vi "QR二维码生成器.vi"(8 "error in (no error)":errorcluster, 9 "timestamp":u64, 10 "signIn":bool, 11 "输入文本":string="殷培\n2013年9月5日\nemail:yin-pei@qq.com") -> (0 "error out":errorcluster, 3 "new picture":picture caption="新图片")   [LabVIEW 2016, in "opSignIn.lvlib"]
uses:
  opSignIn.lvlib
  <vilib>/Utility/miscctls.llb/LVBoundsTypeDef.ctl
panel:
  in  "backcolor":u32(colorbox)=16777215
  in  "color":u32(colorbox)
  in  "掩模图形":u16(ring) items=["000", "001", "010", "011", "100", "101", "110", "111"]
  in  "纠错等级":u16(ring)=2 items=["L(7%)", "M(15%)", "Q(25%)", "H(30%)"]
  in  "版本":u16(ring)=1 items=["1"=1, "2"=2, "3"=3, "4"=4, "5"=5, "6"=6, "7"=7, "8"=8, "9"=9, "10"=10, "11"=11, "12"=12, "13"=13, "14"=14, "15"=15, "16"=16, "17"=17, "18"=18, "19"=19, "20"=20, "21"=21, "22"=22, "23"=23, "24"=24, "25"=25, "26"=26, "27"=27, "28"=28, "29"=29, "30"=30, "31"=31, "32"=32, "33"=33, "34"=34, "35"=35, "36"=36, "37"=37, "38"=38, "39"=39, "40"=40]
  in  "自动？":enum16{"禁止自适应版本", "自适应版本"}(ring)=enum."自适应版本"
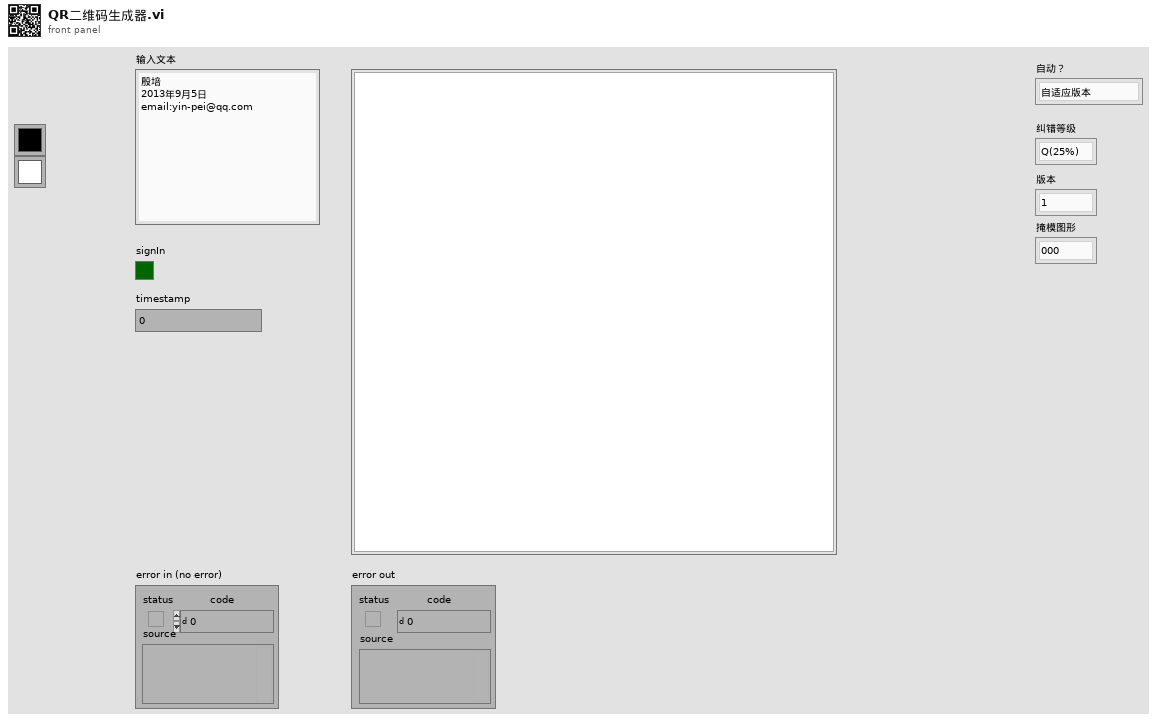
[diagram p1: front panel]
types:
  T1 = typedef "LVBoundsTypeDef.ctl" = cluster{"Width":u32, "Height":u32}
  T2 = cluster{"horizontal":enum16{"left", "center", "right"}, "vertical":enum16{"top", "center", "bottom"}}
  T3 = cluster{"Font Name:":string, "Size":i16, "Strikeout?":bool, "Italic?":bool, "Underline?":bool, "Outline?":bool, "Shadow?":bool, "Bold?":bool}
  T4 = enum16{"User-specified Font", "Application Font", "System Font", "Dialog Font"}
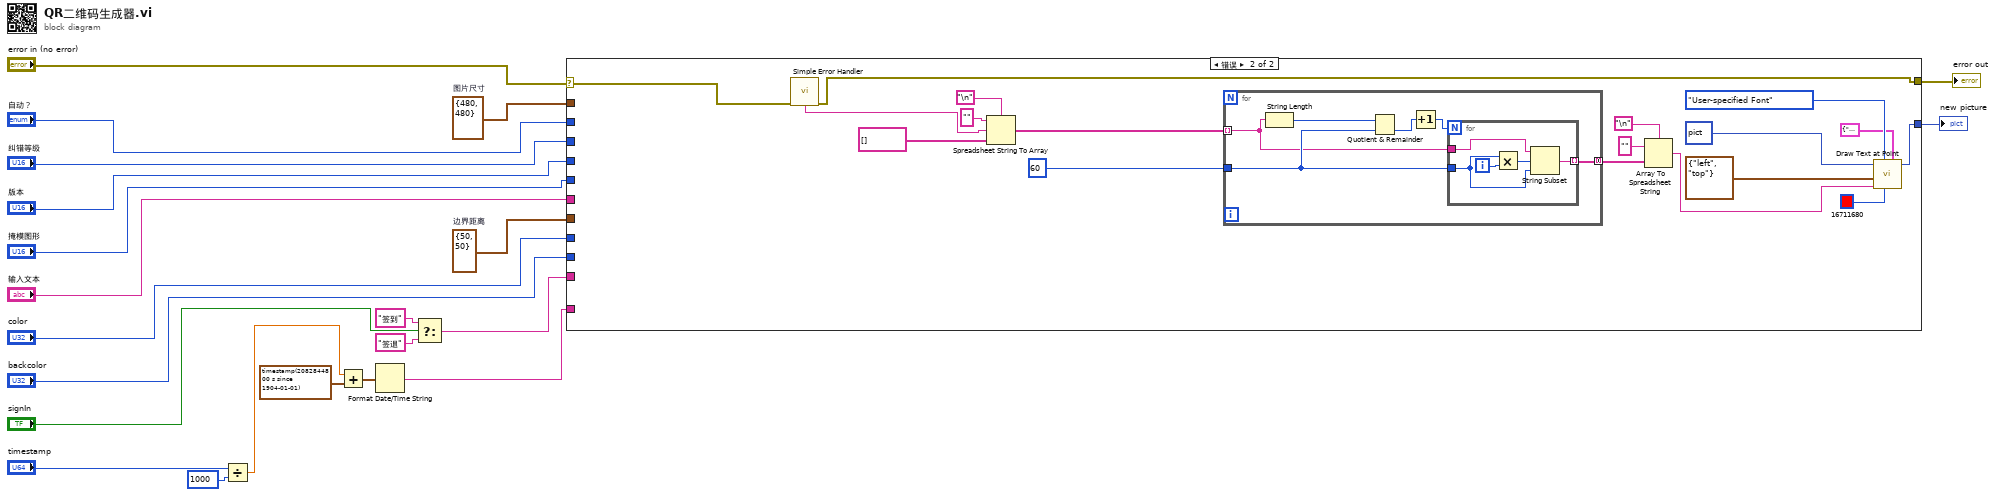
[diagram p0: block diagram]
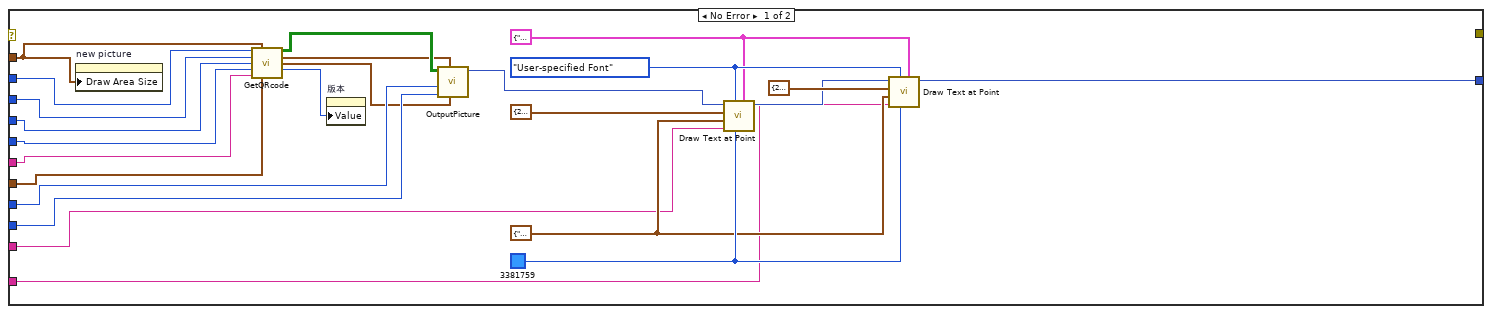
[diagram p2: hidden frame]
diagram:
  w21 = cluster{"x":i16, "y":i16} {"x"=50, "y"=50}  # 边界距离
  w22 = T1 {"Width"=480, "Height"=480}  # 图片尺寸
  n1 = Divide(x="timestamp", y=u64 1000) -> (x/y=w6:dbl)
  n2 = Add(x=w6, y=timestamp(2082844800 s since 1904-01-01)) -> (x+y=w8:timestamp)
  n3 = Format Date/Time String(seconds (now)=w8) -> (date/time string=w2:string)  [unwired: 2 in]
  n4 = Select(t="签到", s="signIn", f="签退") -> (s? t:f=w1:string)
  n5 = case shown="错误" "error in (no error)" {
    selector: "error in (no error)" -> [_ w63]
    tunnel: w22 -> [w46 _]
    tunnel: w21 -> [w45 _]
    tunnel: "backcolor" -> [w44 _]
    tunnel: "color" -> [w43 _]
    tunnel: [w25 w64] -> w11
    tunnel: "输入文本" -> [w42 _]
    tunnel: "掩模图形" -> [w41 _]
    tunnel: "纠错等级" -> [w40 _]
    tunnel: "版本" -> [w39 _]
    tunnel: "自动？" -> [w38 _]
    tunnel: [_ w62] -> w12
    tunnel: w1 -> [w24 _]
    tunnel: w2 -> [w23 _]
    frame No Error {
      w33 = u32 3381759 ("text color(black)")
      w31 = T3 {"Font Name:"="微软雅黑", "Size"=36, "Strikeout?"=FALSE, "Italic?"=FALSE, "Underline?"=FALSE, "Outline?"=FALSE, "Shadow?"=FALSE, "Bold?"=FALSE} ("[user-specified font]")
      w32 = T4."User-specified Font" ("desired font(Application)")
      w29 = T2 {"horizontal"=enum."center", "vertical"=enum."center"} ("alignment(left, top)")
      n6 = property on="new picture" class="Pict"("Draw Area Size"=w46) -> ()  [unwired: 2 in, 2 out]
      n7 = call "GetQRcode.vi"("自动？"=w38, "图片尺寸"=w46, "纠错等级"=w40, "版本"=w39, "掩模图形"=w41, "输入文本"=w42, "边界距离"=w45) -> ("二维码"=w37:bool[][], "显示起点"=w36:cluster{dbl, dbl}, "像素大小"=w35:cluster{dbl, dbl}, "扩展版本"=w34:i32)  [unwired: 5 in]
      n8 = property on="版本" class="Ring (严格)"("Value"=w34) -> ()  [unwired: 2 in, 2 out]
      n9 = call "OutputPicture.vi"("像素大小"=w35, "显示起点"=w36, "backcolor"=w44, "color"=w43, "二维码"=w37) -> ("new picture"=w26:picture)  [unwired: 6 in]
      n10 = call <vilib>:"Draw Text at Point.vi"("[user-specified font]"=w31, "text color(black)"=w33, "desired font(Application)"=w32, "text"=w24, "alignment(left, top)"=w29, "origin"=cluster{"x":i16, "y":i16} {"x"=240, "y"=20}, "picture"=w26) -> ("new picture"=w28:picture)  [unwired: 3 in, 1 out]
      n11 = call <vilib>:"Draw Text at Point.vi"("[user-specified font]"=w31, "text color(black)"=w33, "desired font(Application)"=w32, "text"=w23, "alignment(left, top)"=w29, "origin"=cluster{"x":i16, "y":i16} {"x"=240, "y"=460}, "picture"=w28) -> ("new picture"=w25:picture)  [unwired: 3 in, 1 out]
    }
    frame Error {
      n12 = call <vilib>:"Simple Error Handler.vi"("error in (no error)"=w63) -> ("error out"=w62:errorcluster, "message"=w57:string)  [unwired: 4 in, 3 out]
      n13 = Spreadsheet String To Array(delimiter (Tab)="\n", format string="" ("格式字符串"), spreadsheet string=w57, array type (2D Dbl)=string[] []) -> (array=w56:string[])
      n14 = for {
        tunnel: w56 -> [w65] mode=indexing
        tunnel: 60 ("y") -> [w67]
        tunnel: [w66] -> w50 mode=concatenating
        n15 = String Length(string=w65) -> (length=w70:i32)
        n16 = Quotient & Remainder(x=w70, y=w67) -> (floor(x/y)=w69:i32)  [unwired: 1 out]
        n17 = Increment(x=w69) -> (x+1=w68:i32)
        n18 = for {
          N: w68 -> [_]
          tunnel: w65 -> [w75]
          tunnel: w67 -> [w73]
          tunnel: [w71] -> w66 mode=indexing
          i -> [w74]
          n19 = Multiply(x=w73, y=w74) -> (x*y=w72:i32)
          n20 = String Subset(string=w75, offset (0)=w72, length (rest)=w73) -> (substring=w71:string)
        }
      }
      n21 = Array To Spreadsheet String(delimiter (Tab)="\n", array=w50, 3:"" ("格式字符串")) -> (spreadsheet string=w47:string)
      n22 = call <vilib>:"Draw Text at Point.vi"("[user-specified font]"=T3 {"Font Name:"="微软雅黑", "Size"=17, "Strikeout?"=FALSE, "Italic?"=FALSE, "Underline?"=FALSE, "Outline?"=FALSE, "Shadow?"=FALSE, "Bold?"=FALSE}, "text color(black)"=u32 16711680, "desired font(Application)"=T4."User-specified Font", "text"=w47, "alignment(left, top)"=T2 {"horizontal"=enum."left", "vertical"=enum."top"}, "picture"=picture data[5B] ("new picture")) -> ("new picture"=w64:picture)  [unwired: 4 in, 1 out]
    }
  }
  "new picture" <- w11
  "error out" <- w12
